vi "Mandar.vi"() -> ()   [LabVIEW 2020]
uses:
  <vilib>/httpClient/PUTBuffer.vi
  <vilib>/httpClient/LabVIEWHTTPClient.lvlib
panel:
  in  "stop":bool
  out "error out":errorcluster
  out "body":string
  out "headers":string
  in  "Rele":bool
  in  "Acionamiento":dbl(knob) scale=0.0..10.0
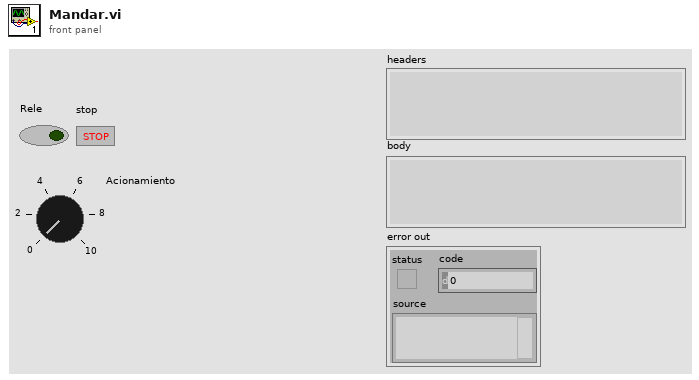
[diagram p1: front panel]
types:
  T1 = cluster{"Acionamiento":dbl, "Data":string, "Hora":string, "Rele":bool}
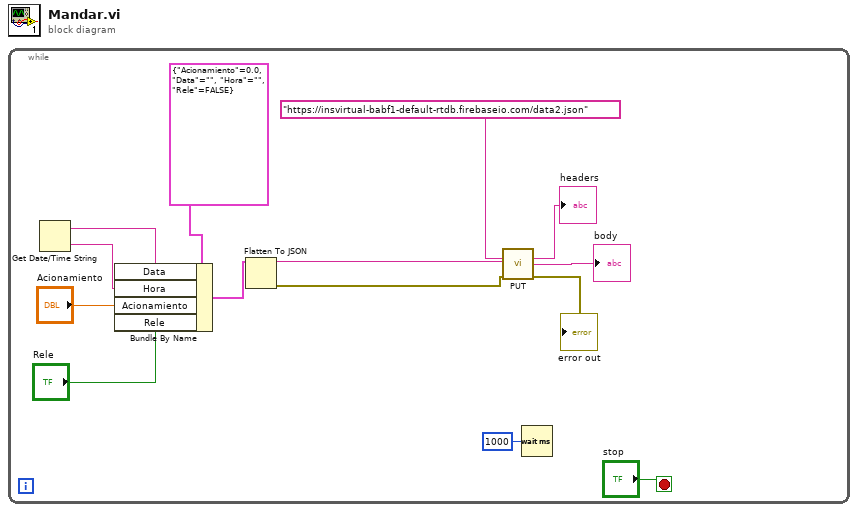
[diagram p0: block diagram]
diagram:
  n1 = while {
    stop <- "stop" stop-if-true
    n2 = Get Date/Time String() -> (date string=w2:string, time string=w1:string)  [unwired: 3 in]
    n3 = Bundle By Name(cluster=T1 {"Acionamiento"=0.0, "Data"="", "Hora"="", "Rele"=FALSE}, "Data"=w2, "Hora"=w1, "Acionamiento"="Acionamiento", "Rele"="Rele") -> (w12:T1)
    n4 = Flatten To JSON(anything=w12) -> (JSON string=w9:string, 11:w8:errorcluster)  [unwired: 2 in]
    n5 = call-poly <vilib>:"PUT.vi"("url"="https://insvirtual-babf1-default-rtdb.firebaseio.com/data2.json", "buffer"=w9, "error in (no error)"=w8) -> ("headers"=→"headers":string, "body"=→"body":string, "error out"=→"error out":errorcluster)  [unwired: 9 in, 1 out]
    n6 = Wait (ms)(milliseconds to wait=u32 1000) -> ()  [unwired: 1 out]
  }
